vi "PID_VI_edits_feb9Copy.vi"(4 "Cooling range?":bool, 5 "Integral allowed?":bool, 6 "output range":cluster{"output high":dbl, "output low":dbl}={"output high"=100.0, "output low"=-100.0} {"output low" format="%.2f"; "output high" format="%.2f"}, 7 "PID gains":T1={"proportional gain (Kc)"=1.0, "integral time (Ti, min)"=0.01, "derivative time (Td, min)"=0.0} {"derivative time (Td, min)" format="%.3f"; "integral time (Ti, min)" format="%.3f"; "proportional gain (Kc)" format="%.3f"}, 8 "dt (s)":dbl=-1.0 format="%.3f", 9 "reinitialize? (F)":bool, 10 "process variable":dbl format="%.2f", 11 "setpoint":dbl format="%.2f") -> (0 "dt out (s)":dbl format="%.3f", 1 "output":dbl format="%.2f", 2 "Integrated error":dbl)   [LabVIEW 2019]
uses:
  Global 9.vi
panel:
  out "initialized array":dbl[](array[numeric])
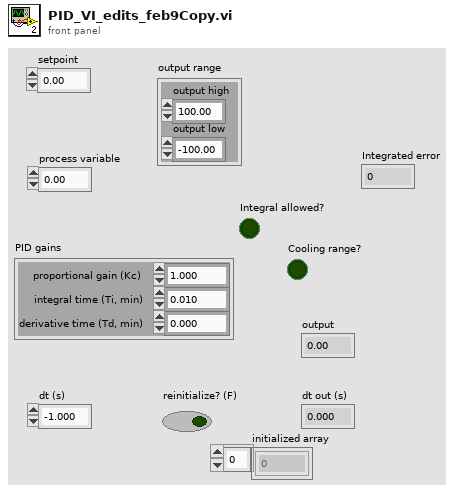
[diagram p1: front panel]
types:
  T1 = cluster{"proportional gain (Kc)":dbl, "integral time (Ti, min)":dbl, "derivative time (Td, min)":dbl}
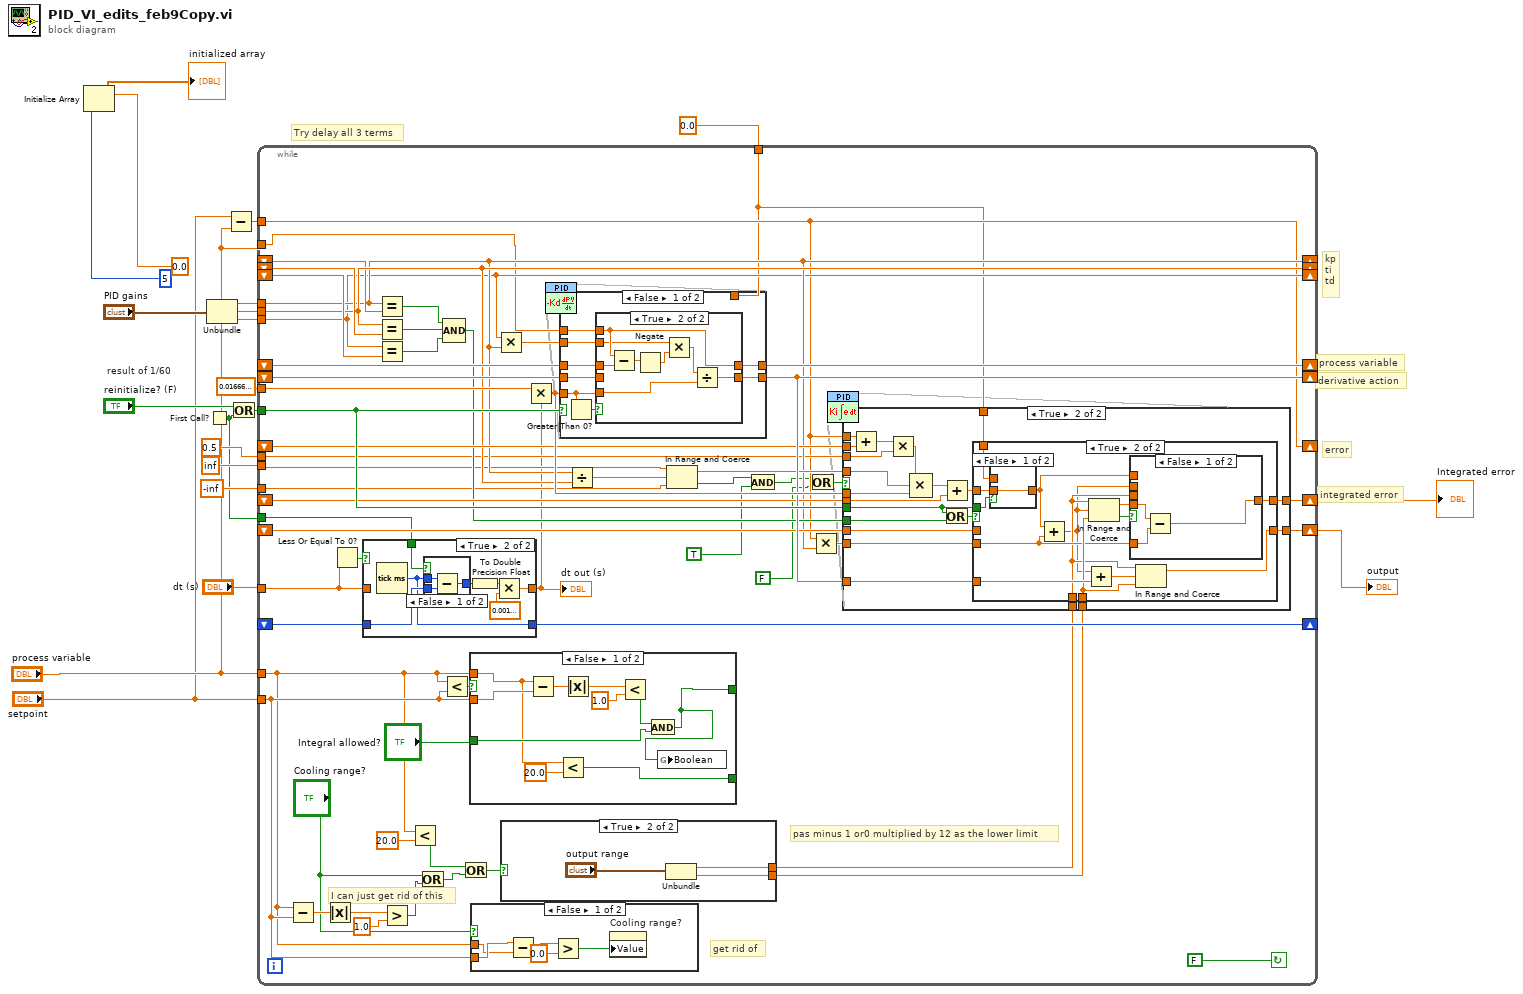
[diagram p0: block diagram]
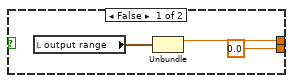
[diagram p3: hidden frame]
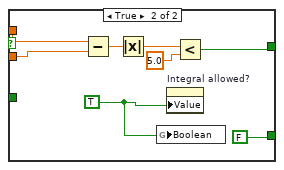
[diagram p4: hidden frame]
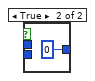
[diagram p6: hidden frame]
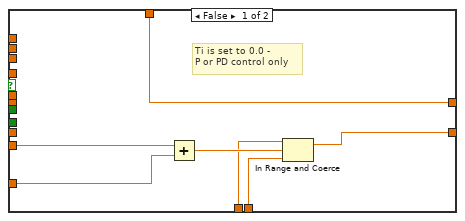
[diagram p7: hidden frame]
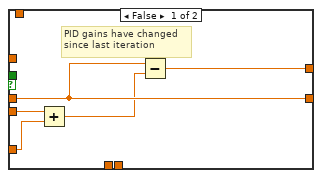
[diagram p8: hidden frame]
diagram:
  w17 = 0.016666666666666666  # result of 1/60
  # "Try delay all 3 terms"
  # "derivative action"
  # "process variable"
  # "kp\nti\ntd"
  # "error"
  # "integrated error"
  n1 = Initialize Array(0.0 ("element"), 5 ("dimension size")) -> (→"initialized array":dbl[])
  n2 = First Call?() -> (First Call?: T/F=w8:bool)
  n3 = Unbundle("PID gains") -> ("proportional gain (Kc)"=w20:dbl, "integral time (Ti, min)"=w19:dbl, "derivative time (Td, min)"=w18:dbl)
  n4 = Subtract(x="setpoint", y="process variable") -> (x-y=w10:dbl)
  n5 = Or(x="reinitialize? (F)", y=w8) -> (x .or. y?=w21:bool)
  n6 = while {
    tunnel: w21 -> [w80]
    shift-left: _ -> [w46]
    shift-right: [w47] -> _
    shift-right: [w56] -> _
    shift-left: _ -> [w57]
    shift-right: [w58] -> _
    shift-left: _ -> [w77]
    shift-right: [w51] -> _
    shift-left: _ -> [w78]
    tunnel: w20 -> [w56]
    tunnel: w19 -> [w58]
    tunnel: w18 -> [w51]
    tunnel: "dt (s)" -> [w45]
    tunnel: "process variable" -> [w25]
    shift-right: [w73] -> _
    shift-left: _ -> [w72]
    shift-right: [w71] -> _
    shift-left: _ -> [w64]
    shift-right: [w70] -> w7
    shift-left: _ -> [w69]
    shift-right: [w50] -> _
    shift-left: _ -> [w68]
    shift-right: [w67] -> w3
    shift-left: _ -> [w66]
    tunnel: w17 -> [w61]
    tunnel: 0.5 ("y") -> [w55]
    tunnel: inf ("upper limit") -> [w53]
    tunnel: -inf ("lower limit") -> [w54]
    tunnel: w10 -> [w50]
    tunnel: 0.0 -> [w49]
    tunnel: w8 -> [w43]
    tunnel: "process variable" -> [w32]
    tunnel: "setpoint" -> [w35]
    stop <- FALSE continue-if-true
    # "get rid of"
    # "I can just get rid of this"
    # "pas minus 1 or0 multiplied by 12 as the lower limit"
    n7 = Subtract(x=w32, y=w35) -> (x-y=w38:dbl)
    n8 = Absolute Value(x=w38) -> (abs(x)=w37:dbl)
    n9 = Less Or Equal To 0?(x=w45) -> (x <= 0?=w44:bool)
    n10 = case shown="True" w44 {
      tunnel: [w111 w115] -> w48
      tunnel: w46 -> [w110 w114]
      tunnel: [w110 w113] -> w47
      tunnel: w45 -> [w111 _]
      tunnel: w43 -> [_ w112]
      frame False {
      }
      frame True {
        n11 = Tick Count (ms)() -> (millisecond timer value=w113:u32)
        n12 = case shown="False" w112 {
          tunnel: [w121 u32 0] -> w117
          tunnel: w114 -> [w120 _]
          tunnel: w113 -> [w119 _]
          frame False {
            n13 = Subtract(x=w119, y=w120) -> (x-y=w121:u32)
          }
          frame True {
          }
        }
        n14 = To Double Precision Float(number=w117) -> (double precision float=w116:dbl)
        n15 = Multiply(x=w116, y=0.0010000000474974513) -> (x*y=w115:dbl)
      }
    }
    "dt out (s)" <- w48
    n16 = Equal?(x=w56, y=w57) -> (x = y?=w75:bool)
    n17 = Equal?(x=w58, y=w77) -> (x = y?=w74:bool)
    n18 = Equal?(x=w51, y=w78) -> (x = y?=w76:bool)
    n19 = Greater?(x=w37, y=1.0) -> (0:w26:bool)
    n20 = Less?(x=w32, y=20.0) -> (x < y?=w33:bool)
    n21 = Or(x="Cooling range?", y=w26) -> (x .or. y?=w27:bool)
    n22 = Less?(x=w32, y=w35) -> (x < y?=w41:bool)
    n23 = Compound Arithmetic op=AND(w75, w74, w76) -> (w59:bool)
    n24 = Or(x=w33, y=w27) -> (x .or. y?=w28:bool)
    n25 = case shown="False" w41 {
      tunnel: [w95 w108] -> _
      tunnel: w32 -> [w94 w107]
      tunnel: w35 -> [w98 w106]
      tunnel: "Integral allowed?" -> [w96 _]
      tunnel: [w92 FALSE] -> _
      frame False {
        n26 = Subtract(x=w94, y=w98) -> (x-y=w101:dbl)
        n27 = Less?(x=w94, y=20.0) -> (x < y?=w92:bool)
        n28 = Absolute Value(x=w101) -> (abs(x)=w100:dbl)
        n29 = Less?(x=w100, y=1.0) -> (x < y?=w97:bool)
        n30 = And(x=w97, y=w96) -> (x .and. y?=w95:bool)
        n31 = global write "Global 9.vi" "Boolean"(w95) -> ()
      }
      frame True {
        w103 = TRUE
        n32 = Subtract(x=w107, y=w106) -> (x-y=w105:dbl)
        n33 = Absolute Value(x=w105) -> (abs(x)=w104:dbl)
        n34 = global write "Global 9.vi" "Boolean"(w103) -> ()
        n35 = property on="Integral allowed?" class="Bool (strict)"("Value"=w103) -> ()  [unwired: 2 in, 2 out]
        n36 = Less?(x=w104, y=5.0) -> (x < y?=w108:bool)
      }
    }
    n37 = case shown="False" "Cooling range?" {
      tunnel: w32 -> [w84 _]
      tunnel: w35 -> [w85 _]
      frame False {
        n38 = Subtract(x=w85, y=w84) -> (x-y=w83:dbl)
        n39 = Greater?(x=w83, y=0.0) -> (0:w81:bool)
        n40 = property on="Cooling range?" class="Bool (strict)"("Value"=w81) -> ()  [unwired: 2 in, 2 out]
      }
      frame True {
      }
    }
    n41 = Multiply(x=w51, y=w56) -> (x*y=w63:dbl)
    n42 = case shown="True" w28 {
      tunnel: [w88 w90] -> w40
      tunnel: [0.0 ("output low") w89] -> w39
      frame False {
        n43 = local read "output range"() -> (w86:cluster{"output high":dbl, "output low":dbl})
        n44 = Unbundle(w86) -> ("output high"=w88:dbl)  [unwired: 1 out]
      }
      frame True {
        n45 = Unbundle("output range") -> ("output high"=w90:dbl, "output low"=w89:dbl)
      }
    }
    n46 = Multiply(x=w61, y=w48) -> (x*y=w79:dbl)
    n47 = case shown="False" w80 {
      tunnel: w72 -> [w183 _]
      tunnel: w63 -> [w180 _]
      tunnel: w25 -> [w182 w195]
      tunnel: [w179 w195] -> w73
      tunnel: [w181 w194] -> w71
      tunnel: w64 -> [w177 _]
      tunnel: w79 -> [w176 _]
      tunnel: w49 -> [_ w194]
      frame False {
        n48 = Greater Than 0?(x=w176) -> (x > 0?=w178:bool)
        n49 = case shown="True" w178 {
          tunnel: w183 -> [w185 w191]
          tunnel: w176 -> [_ w190]
          tunnel: w182 -> [_ w188]
          tunnel: [w184 w189] -> w181
          tunnel: w180 -> [_ w186]
          tunnel: [w185 w188] -> w179
          tunnel: w177 -> [w184 _]
          frame False {
            # "dt = 0 min"
          }
          frame True {
            n50 = Subtract(x=w188, y=w191) -> (x-y=w193:dbl)
            n51 = Negate(x=w193) -> (-x=w187:dbl)
            n52 = Multiply(x=w186, y=w187) -> (x*y=w192:dbl)
            n53 = Divide(x=w192, y=w190) -> (x/y=w189:dbl)
          }
        }
      }
      frame True {
      }
    }
    n54 = Divide(x=w56, y=w58) -> (x/y=w62:dbl)
    n55 = In Range and Coerce(upper limit=w53, x=w62, lower limit=w54) -> (coerced(x)=w65:dbl, In Range?=w42:bool)
    n56 = And(x=w42, y=TRUE) -> (x .and. y?=w30:bool)
    n57 = Or(x=w30, y=FALSE) -> (x .or. y?=w29:bool)
    n58 = Multiply(x=w50, y=w56) -> (x*y=w60:dbl)
    n59 = case shown="True" w29 {
      tunnel: w50 -> [_ w149]
      tunnel: w68 -> [_ w150]
      tunnel: w66 -> [_ w145]
      tunnel: [w123 w140] -> w67
      tunnel: w65 -> [_ w138]
      tunnel: w60 -> [w128 w143]
      tunnel: [w129 w139] -> w70
      tunnel: w69 -> [_ w141]
      tunnel: w71 -> [w127 w137]
      tunnel: w80 -> [_ w136]
      tunnel: w59 -> [_ w135]
      tunnel: w79 -> [_ w134]
      tunnel: w40 -> [w125 w132]
      tunnel: w39 -> [w124 w133]
      tunnel: w55 -> [_ w131]
      tunnel: w49 -> [w123 w130]
      frame False {
        # "Ti is set to 0.0 -\nP or PD control only"
        n60 = Add(x=w128, y=w127) -> (x+y=w126:dbl)
        n61 = In Range and Coerce(upper limit=w125, x=w126, lower limit=w124) -> (coerced(x)=w129:dbl)  [unwired: 1 out]
      }
      frame True {
        n62 = Add(x=w149, y=w150) -> (x+y=w148:dbl)
        n63 = Multiply(x=w148, y=w131) -> (x*y=w147:dbl)
        n64 = Compound Arithmetic op=MULTIPLY(w147, w138, w134) -> (w146:dbl)
        n65 = Add(x=w146, y=w145) -> (x+y=w144:dbl)
        n66 = Or(x=w136, y=w135) -> (x .or. y?=w142:bool)
        n67 = case shown="True" w142 {
          tunnel: w144 -> [_ w163]
          tunnel: w143 -> [w153 w158]
          tunnel: w141 -> [w155 _]
          tunnel: w136 -> [_ w165]
          tunnel: [w154 w160] -> w140
          tunnel: [w155 w168] -> w139
          tunnel: w137 -> [w152 w167]
          tunnel: w133 -> [_ w166]
          tunnel: w132 -> [_ w157]
          tunnel: w130 -> [_ w164]
          frame False {
            # "PID gains have changed\nsince last iteration"
            n68 = Add(x=w153, y=w152) -> (x+y=w151:dbl)
            n69 = Subtract(x=w155, y=w151) -> (x-y=w154:dbl)
          }
          frame True {
            n70 = case shown="False" w165 {
              tunnel: w164 -> [_ w175]
              tunnel: [w174 w175] -> w162
              tunnel: w163 -> [w174 _]
              frame False {
              }
              frame True {
              }
            }
            n71 = Add(x=w162, y=w158) -> (x+y=w156:dbl)
            n72 = Add(x=w156, y=w167) -> (x+y=w169:dbl)
            n73 = In Range and Coerce(upper limit=w157, x=w156, lower limit=w166) -> (coerced(x)=w159:dbl, In Range?=w161:bool)
            n74 = case shown="False" w161 {
              tunnel: w162 -> [_ w173]
              tunnel: [w170 w173] -> w160
              tunnel: w159 -> [w172 _]
              tunnel: w158 -> [w171 _]
              tunnel: w157 -> [_ _]
              tunnel: w156 -> [_ _]
              frame False {
                n75 = Subtract(x=w172, y=w171) -> (x-y=w170:dbl)
              }
              frame True {
              }
            }
            n76 = In Range and Coerce(upper limit=w157, x=w169, lower limit=w166) -> (coerced(x)=w168:dbl)  [unwired: 1 out]
          }
        }
      }
    }
  }
  "output" <- w7
  "Integrated error" <- w3
